vi "Modificación_Arreglos_Recetas.vi"(9 "Recetas In":T1 {"Recetas LS Electric"."Modbus LS-Electric"."Delay respuesta" min=1 max=250 format="%.0f mseg."; "Recetas LS Electric"."Modbus LS-Electric"."Formato RS485" items=["RTU 8-N-1", "RTU 8-N-2", "RTU 8-E-1", "RTU 8-O-1"]; "Recetas LS Electric"."Modbus LS-Electric"."Velocidad datos" items=["1200 bps", "2400 bps", "4800 bps", "9600 bps", "19200 bps", "38400 bps", "56 kbps", "115 kbps"]; "Recetas LS Electric"."Modbus LS-Electric"."Identificador" min=1 max=250; "Recetas LS Electric"."Motor LS-Electric 2"."Voltaje nominal" min=170 max=480 format="%.0f V"; "Recetas LS Electric"."Motor LS-Electric 2"."Potencia nominal" items=["0.2 kW", "0.4 kW", "0.75 kW", "1.1 kW", "1.5 kW", "2.2 kW", "3.0 kW", "3.7 kW", "4.0 kW", "5.5 kW", "7.5 kW", "11.kW"]; "Recetas LS Electric"."Motor LS-Electric 2"."T. Desaceleración" format="%#_g seg"; "Recetas LS Electric"."Motor LS-Electric 2"."T. Aceleración" format="%#_g seg"; "Recetas LS Electric"."Motor LS-Electric 2"."Frecuencia máxima" format="%#_g Hz"; "Recetas LS Electric"."Motor LS-Electric 2"."Frecuencia mínima" format="%#_g Hz"; "Recetas LS Electric"."Motor LS-Electric 2"."Polos" min=2 max=48; "Recetas LS Electric"."Motor LS-Electric 2"."Velocidad nominal" format="%.0f rpm"; "Recetas LS Electric"."Motor LS-Electric 2"."Corriente nominal" format="%#_g Amp"; "Recetas LS Electric"."Motor LS-Electric 2"."Corriente sin carga" format="%#_g Amp"; "Recetas LS Electric"."Motor LS-Electric 2"."Frecuencia nominal" items=["60 Hz", "50 Hz"]; "Recetas LS Electric"."Referencias LS-Electric"."Referencia velocidad 2" items=["No asignar"=0, "Analógica (AI1)"=1, "Analógica (AI2)"=2, "Analógica (AI3)"=3, "Modbus"=164, "Potenciómetro (AIU1)"=183]; "Recetas LS Electric"."Referencias LS-Electric"."Referencia arranque 2" items=["Terminales"=1, "Modbus"=10]; "Recetas LS Electric"."Referencias LS-Electric"."Referencia velocidad 1" items=["No asignar"=0, "Analógica (AI1)"=1, "Analógica (AI2)"=2, "Analógica (AI3)"=3, "Modbus"=164, "Potenciómetro (AIU1)"=183]; "Recetas LS Electric"."Referencias LS-Electric"."Referencia arranque 1" items=["Terminales"=1, "Modbus"=10]; "Recetas LS Electric"."I/O LS-Electric"."Relevador 2" items=["Modbus"=0, "FDT-1"=1, "FDT-2"=2, "FDT-3"=3, "FDT-4"=4, "Sobrecarga"=5, "Sobrevoltaje"=10, "Bajo voltaje"=11, "Sobrecalentamiento"=12, "RUN"=14, "STOP"=15, "Listo"=22]; "Recetas LS Electric"."I/O LS-Electric"."Relevador 1" items=["Modbus"=0, "FDT-1"=1, "FDT-2"=2, "FDT-3"=3, "FDT-4"=4, "Sobrecarga"=5, "Sobrevoltaje"=10, "Bajo voltaje"=11, "Sobrecalentamiento"=12, "RUN"=14, "STOP"=15, "Listo"=22]; "Recetas LS Electric"."I/O LS-Electric"."Entrada 5 (P5)" items=["No asignar"=0, "FWD"=1, "REV"=2, "Reset"=3, "Fallo auxiliar (BX)"=5, "Habilitar RUN"=13, "3 hilos"=14, "Segunda referencia"=15, "Segundo motor"=26]; "Recetas LS Electric"."I/O LS-Electric"."Entrada 4 (P4)" items=["Sin asignar"=0, "FWD"=1, "REV"=2, "Reset"=3, "Fallo auxiliar (BX)"=5, "Habilitar RUN"=13, "3 hilos"=14, "Segunda referencia"=15, "Segundo motor"=26]; "Recetas LS Electric"."I/O LS-Electric"."Entrada 3 (P3)" items=["No asignar"=0, "FWD"=1, "REV"=2, "Reset"=3, "Fallo auxiliar (BX)"=5, "Habilitar RUN"=13, "3 hilos"=14, "Segunda referencia"=15, "Segundo motor"=26]; "Recetas LS Electric"."I/O LS-Electric"."Entrada 2 (P2)" items=["No asignar"=0, "FWD"=1, "REV"=2, "Reset"=3, "Fallo auxiliar (BX)"=5, "Habilitar RUN"=13, "3 hilos"=14, "Segunda referencia"=15, "Segundo motor"=26]; "Recetas LS Electric"."I/O LS-Electric"."Entrada 1 (P1)" items=["No asignar"=0, "FWD"=1, "REV"=2, "Reset"=3, "Fallo auxiliar (BX)"=5, "Habilitar RUN"=13, "3 hilos"=14, "Segunda referencia"=15, "Segundo motor"=26]; "Recetas ABB"."Referencias ABB"."Referencia velocidad 2" items=["No asignar"=0, "Analógica (AI1)"=1, "Analógica (AI2)"=2, "Analógica (AI3)"=3, "Modbus"=164, "Potenciómetro (AIU1)"=183]; "Recetas ABB"."Referencias ABB"."Referencia arranque 2" items=["Terminales"=1, "Modbus"=10]; "Recetas ABB"."Referencias ABB"."Referencia velocidad 1" items=["No asignar"=0, "Analógica (AI1)"=1, "Analógica (AI2)"=2, "Analógica (AI3)"=3, "Modbus"=164, "Potenciómetro (AIU1)"=183]; "Recetas ABB"."Referencias ABB"."Referencia arranque 1" items=["Terminales"=1, "Modbus"=10]; "Recetas ABB"."I/O ABB"."Entrada 4 (DI4)" items=["Sin asignar"=0, "Referencia vel. 2"=1, "Referencia vel. 3"=2, "Fallo auxiliar"=12, "Reset"=13, "Entrada lógica 1"=24, "Entrada lógica 2"=25]; "Recetas ABB"."I/O ABB"."Entrada 3 (DI3)" items=["No asignar"=0, "Referencia vel. 2"=1, "Referencia vel. 3"=2, "Fallo auxiliar"=12, "Reset"=13, "Entrada lógica 1"=24, "Entrada lógica 2"=25]; "Recetas ABB"."I/O ABB"."Entrada 2 (DI2)" items=["No asignar"=0, "Referencia vel. 2"=1, "Referencia vel. 3"=2, "Fallo auxiliar"=12, "Reset"=13, "Entrada lógica 1"=24, "Entrada lógica 2"=25, "REV 2 hilos"=50, "DIR 3 hilos"=51]; "Recetas ABB"."I/O ABB"."Entrada 1 (DI1)" items=["No asignar"=0, "Referencia vel. 2"=1, "Referencia vel. 3"=2, "Fallo auxiliar"=12, "Reset"=13, "Entrada lógica 1"=24, "Entrada lógica 2"=25, "FWD 2 hilos"=48, "RUN 3 hilos"=49]; "Recetas Delta"."Referencias Delta"."Referencia velocidad 2" items=["No asignar"=0, "Analógica (AI1)"=1, "Analógica (AI2)"=2, "Analógica (AI3)"=3, "Modbus"=164, "Potenciómetro (AIU1)"=183]; "Recetas Delta"."Referencias Delta"."Referencia arranque 2" items=["Terminales"=1, "Modbus"=10]; "Recetas Delta"."Referencias Delta"."Referencia velocidad 1" items=["No asignar"=0, "Analógica (AI1)"=1, "Analógica (AI2)"=2, "Analógica (AI3)"=3, "Modbus"=164, "Potenciómetro (AIU1)"=183]; "Recetas Delta"."Referencias Delta"."Referencia arranque 1" items=["Terminales"=1, "Modbus"=10]; "Recetas Delta"."I/O Delta"."Entrada 6 (MI6)" items=["Listo/Fallo"=0, "A frecuencia"=1, "Alimentación"=2, "Sobrefrecuencia"=6, "Sobrecorriente"=7, "Sobretensión"=8, "Modbus"=13]; "Recetas Delta"."I/O Delta"."Entrada 5 (MI5)" items=["Listo/Fallo"=0, "A frecuencia"=1, "Alimentación"=2, "Sobrefrecuencia"=6, "Sobrecorriente"=7, "Sobretensión"=8, "Modbus"=13]; "Recetas Delta"."I/O Delta"."Entrada 4 (MI4)" items=["Sin asignar"=0, "Referencia vel. 2"=1, "Referencia vel. 3"=2, "Fallo auxiliar"=12, "Reset"=13, "Entrada lógica 1"=24, "Entrada lógica 2"=25]; "Recetas Delta"."I/O Delta"."Entrada 3 (MI3)" items=["No asignar"=0, "Referencia vel. 2"=1, "Referencia vel. 3"=2, "Fallo auxiliar"=12, "Reset"=13, "Entrada lógica 1"=24, "Entrada lógica 2"=25]; "Recetas Delta"."I/O Delta"."Entrada 2 (MI2)" items=["No asignar"=0, "Referencia vel. 2"=1, "Referencia vel. 3"=2, "Fallo auxiliar"=12, "Reset"=13, "Entrada lógica 1"=24, "Entrada lógica 2"=25, "REV 2 hilos"=50, "DIR 3 hilos"=51]; "Recetas Delta"."I/O Delta"."Entrada 1 (MI1)" items=["No asignar"=0, "Referencia vel. 2"=1, "Referencia vel. 3"=2, "Fallo auxiliar"=12, "Reset"=13, "Entrada lógica 1"=24, "Entrada lógica 2"=25, "FWD 2 hilos"=48, "RUN 3 hilos"=49]; "Recetas Schneider"."I/O Schneider"."Transistor" items=["Listo/Fallo"=0, "A frecuencia"=1, "Alimentación"=2, "Sobrefrecuencia"=6, "Sobrecorriente"=7, "Sobretensión"=8, "Modbus"=13]; "Recetas Schneider"."I/O Schneider"."Relevador 2 (R2)" items=["Listo/Fallo"=0, "A frecuencia"=1, "Alimentación"=2, "Sobrefrecuencia"=6, "Sobrecorriente"=7, "Sobretensión"=8, "Modbus"=13]; "Recetas Schneider"."I/O Schneider"."Relevador 1 (R1)" items=["Listo/Fallo"=0, "A frecuencia"=1, "Alimentación"=2, "Sobrefrecuencia"=6, "Sobrecorriente"=7, "Sobretensión"=8, "Modbus"=13]; "Recetas Schneider"."I/O Schneider"."Entrada 6 (DI6)" items=["Listo/Fallo"=0, "A frecuencia"=1, "Alimentación"=2, "Sobrefrecuencia"=6, "Sobrecorriente"=7, "Sobretensión"=8, "Modbus"=13]; "Recetas Schneider"."I/O Schneider"."Entrada 5 (DI5)" items=["Listo/Fallo"=0, "A frecuencia"=1, "Alimentación"=2, "Sobrefrecuencia"=6, "Sobrecorriente"=7, "Sobretensión"=8, "Modbus"=13]; "Recetas Schneider"."I/O Schneider"."Entrada 4 (DI4)" items=["Sin asignar"=0, "Referencia vel. 2"=1, "Referencia vel. 3"=2, "Fallo auxiliar"=12, "Reset"=13, "Entrada lógica 1"=24, "Entrada lógica 2"=25]; "Recetas Schneider"."I/O Schneider"."Entrada 3 (DI3)" items=["No asignar"=0, "Referencia vel. 2"=1, "Referencia vel. 3"=2, "Fallo auxiliar"=12, "Reset"=13, "Entrada lógica 1"=24, "Entrada lógica 2"=25]; "Recetas Schneider"."I/O Schneider"."Entrada 2 (DI2)" items=["No asignar"=0, "Referencia vel. 2"=1, "Referencia vel. 3"=2, "Fallo auxiliar"=12, "Reset"=13, "Entrada lógica 1"=24, "Entrada lógica 2"=25, "REV 2 hilos"=50, "DIR 3 hilos"=51]; "Recetas Schneider"."I/O Schneider"."Entrada 1 (DI1)" items=["No asignar"=0, "Referencia vel. 2"=1, "Referencia vel. 3"=2, "Fallo auxiliar"=12, "Reset"=13, "Entrada lógica 1"=24, "Entrada lógica 2"=25, "FWD 2 hilos"=48, "RUN 3 hilos"=49]; "Recetas Schneider"."Referencias Schneider"."Referencia velocidad 2" items=["No asignar"=0, "Analógica (AI1)"=1, "Analógica (AI2)"=2, "Analógica (AI3)"=3, "Modbus"=164, "Potenciómetro (AIU1)"=183]; "Recetas Schneider"."Referencias Schneider"."Referencia arranque 2" items=["Terminales"=1, "Modbus"=10]; "Recetas Schneider"."Referencias Schneider"."Referencia velocidad 1" items=["No asignar"=0, "Analógica (AI1)"=1, "Analógica (AI2)"=2, "Analógica (AI3)"=3, "Modbus"=164, "Potenciómetro (AIU1)"=183]; "Recetas Schneider"."Referencias Schneider"."Referencia arranque 1" items=["Terminales"=1, "Modbus"=10]; "Recetas Allen Bradley"."Modbus PowerFlex"."Tmp. pérdida comun." min=0.0 max=60.0 format="%#_g seg."; "Recetas Allen Bradley"."Modbus PowerFlex"."Identificador" min=1 max=247; "Recetas Allen Bradley"."Modbus PowerFlex"."Formato RS485" items=["RTU 8-N-1", "RTU 8-E-1", "RTU 8-O-1", "RTU 8-N-2", "RTU 8-E-2", "RTU 8-O-2"]; "Recetas Allen Bradley"."Modbus PowerFlex"."Acc. pérdida comun." items=["Fallo", "Paro inercia", "Paro", "Nada"]; "Recetas Allen Bradley"."Modbus PowerFlex"."Velocidad datos" items=["9600 bps", "2400 bps", "4800 bps", "9600 bps", "19200 bps", "38400 bps"]; "Recetas Allen Bradley"."Motor PowerFlex"."T. Desaleceración" format="%#_g seg"; "Recetas Allen Bradley"."Motor PowerFlex"."T. Aceleración" format="%#_g seg"; "Recetas Allen Bradley"."Motor PowerFlex"."Velocidad nominal" format="%.0f rpm"; "Recetas Allen Bradley"."Motor PowerFlex"."Voltaje nominal" format="%.0f V"; "Recetas Allen Bradley"."Motor PowerFlex"."Frecuencia nominal" format="%.0f Hz"; "Recetas Allen Bradley"."Motor PowerFlex"."Corriente sobrecarga" format="%#_g Amp"; "Recetas Allen Bradley"."Motor PowerFlex"."Corriente nominal" format="%#_g Amp"; "Recetas Allen Bradley"."Motor PowerFlex"."Polos" min=2 max=40; "Recetas Allen Bradley"."I/O PowerFlex"."Relevador" items=["Listo/Fallo"=0, "A frecuencia"=1, "Alimentación"=2, "Sobrefrecuencia"=6, "Sobrecorriente"=7, "Sobretensión"=8, "Modbus"=13]; "Recetas Allen Bradley"."I/O PowerFlex"."Entrada 6 (06)" items=["No asignar"=0, "Referencia vel. 2"=1, "Referencia vel. 3"=2, "Fallo auxiliar"=12, "Reset"=13, "Entrada lógica 1"=24, "Entrada lógica 2"=25]; "Recetas Allen Bradley"."I/O PowerFlex"."Entrada 5 (05)" items=["No asignar"=0, "Referencia vel. 2"=1, "Referencia vel. 3"=2, "Fallo auxiliar"=12, "Reset"=13, "Entrada lógica 1"=24, "Entrada lógica 2"=25]; "Recetas Allen Bradley"."I/O PowerFlex"."Entrada 3 (03)" items=["No asignar"=0, "Referencia vel. 2"=1, "Referencia vel. 3"=2, "Fallo auxiliar"=12, "Reset"=13, "Entrada lógica 1"=24, "Entrada lógica 2"=25, "REV 2 hilos"=50, "DIR 3 hilos"=51]; "Recetas Allen Bradley"."I/O PowerFlex"."Entrada 2 (02)" items=["No asignar"=0, "Referencia vel. 2"=1, "Referencia vel. 3"=2, "Fallo auxiliar"=12, "Reset"=13, "Entrada lógica 1"=24, "Entrada lógica 2"=25, "FWD 2 hilos"=48, "RUN 3 hilos"=49]; "Recetas Allen Bradley"."Referencias PowerFlex"."Referencia velocidad 2" items=["Potenciómetro"=1, "Teclado"=2, "Modbus"=3, "Analógica (0-10V)"=5, "Analógica (4-20mA)"=6]; "Recetas Allen Bradley"."Referencias PowerFlex"."Referencia arranque 2" items=["Teclado"=1, "Terminales"=2, "Modbus"=3]; "Recetas Allen Bradley"."Referencias PowerFlex"."Referencia velocidad 1" items=["Potenciómetro"=1, "Teclado"=2, "Modbus"=3, "Analógica (0-10V)"=5, "Analógica (4-20mA)"=6]; "Recetas Allen Bradley"."Referencias PowerFlex"."Referencia arranque 1" items=["Teclado"=1, "Terminales"=2, "Modbus"=3]}, 10 "Fabricante":u32, 11 "Índice":u32) -> (3 "Recetas Out":T1 {"Recetas LS Electric"."Modbus LS-Electric"."Delay respuesta" min=1 max=250 format="%.0f mseg."; "Recetas LS Electric"."Modbus LS-Electric"."Formato RS485" items=["RTU 8-N-1", "RTU 8-N-2", "RTU 8-E-1", "RTU 8-O-1"]; "Recetas LS Electric"."Modbus LS-Electric"."Velocidad datos" items=["1200 bps", "2400 bps", "4800 bps", "9600 bps", "19200 bps", "38400 bps", "56 kbps", "115 kbps"]; "Recetas LS Electric"."Modbus LS-Electric"."Identificador" min=1 max=250; "Recetas LS Electric"."Motor LS-Electric 2"."Voltaje nominal" min=170 max=480 format="%.0f V"; "Recetas LS Electric"."Motor LS-Electric 2"."Potencia nominal" items=["0.2 kW", "0.4 kW", "0.75 kW", "1.1 kW", "1.5 kW", "2.2 kW", "3.0 kW", "3.7 kW", "4.0 kW", "5.5 kW", "7.5 kW", "11.kW"]; "Recetas LS Electric"."Motor LS-Electric 2"."T. Desaceleración" format="%#_g seg"; "Recetas LS Electric"."Motor LS-Electric 2"."T. Aceleración" format="%#_g seg"; "Recetas LS Electric"."Motor LS-Electric 2"."Frecuencia máxima" format="%#_g Hz"; "Recetas LS Electric"."Motor LS-Electric 2"."Frecuencia mínima" format="%#_g Hz"; "Recetas LS Electric"."Motor LS-Electric 2"."Polos" min=2 max=48; "Recetas LS Electric"."Motor LS-Electric 2"."Velocidad nominal" format="%.0f rpm"; "Recetas LS Electric"."Motor LS-Electric 2"."Corriente nominal" format="%#_g Amp"; "Recetas LS Electric"."Motor LS-Electric 2"."Corriente sin carga" format="%#_g Amp"; "Recetas LS Electric"."Motor LS-Electric 2"."Frecuencia nominal" items=["60 Hz", "50 Hz"]; "Recetas LS Electric"."Referencias LS-Electric"."Referencia velocidad 2" items=["No asignar"=0, "Analógica (AI1)"=1, "Analógica (AI2)"=2, "Analógica (AI3)"=3, "Modbus"=164, "Potenciómetro (AIU1)"=183]; "Recetas LS Electric"."Referencias LS-Electric"."Referencia arranque 2" items=["Terminales"=1, "Modbus"=10]; "Recetas LS Electric"."Referencias LS-Electric"."Referencia velocidad 1" items=["No asignar"=0, "Analógica (AI1)"=1, "Analógica (AI2)"=2, "Analógica (AI3)"=3, "Modbus"=164, "Potenciómetro (AIU1)"=183]; "Recetas LS Electric"."Referencias LS-Electric"."Referencia arranque 1" items=["Terminales"=1, "Modbus"=10]; "Recetas LS Electric"."I/O LS-Electric"."Relevador 2" items=["Modbus"=0, "FDT-1"=1, "FDT-2"=2, "FDT-3"=3, "FDT-4"=4, "Sobrecarga"=5, "Sobrevoltaje"=10, "Bajo voltaje"=11, "Sobrecalentamiento"=12, "RUN"=14, "STOP"=15, "Listo"=22]; "Recetas LS Electric"."I/O LS-Electric"."Relevador 1" items=["Modbus"=0, "FDT-1"=1, "FDT-2"=2, "FDT-3"=3, "FDT-4"=4, "Sobrecarga"=5, "Sobrevoltaje"=10, "Bajo voltaje"=11, "Sobrecalentamiento"=12, "RUN"=14, "STOP"=15, "Listo"=22]; "Recetas LS Electric"."I/O LS-Electric"."Entrada 5 (P5)" items=["No asignar"=0, "FWD"=1, "REV"=2, "Reset"=3, "Fallo auxiliar (BX)"=5, "Habilitar RUN"=13, "3 hilos"=14, "Segunda referencia"=15, "Segundo motor"=26]; "Recetas LS Electric"."I/O LS-Electric"."Entrada 4 (P4)" items=["Sin asignar"=0, "FWD"=1, "REV"=2, "Reset"=3, "Fallo auxiliar (BX)"=5, "Habilitar RUN"=13, "3 hilos"=14, "Segunda referencia"=15, "Segundo motor"=26]; "Recetas LS Electric"."I/O LS-Electric"."Entrada 3 (P3)" items=["No asignar"=0, "FWD"=1, "REV"=2, "Reset"=3, "Fallo auxiliar (BX)"=5, "Habilitar RUN"=13, "3 hilos"=14, "Segunda referencia"=15, "Segundo motor"=26]; "Recetas LS Electric"."I/O LS-Electric"."Entrada 2 (P2)" items=["No asignar"=0, "FWD"=1, "REV"=2, "Reset"=3, "Fallo auxiliar (BX)"=5, "Habilitar RUN"=13, "3 hilos"=14, "Segunda referencia"=15, "Segundo motor"=26]; "Recetas LS Electric"."I/O LS-Electric"."Entrada 1 (P1)" items=["No asignar"=0, "FWD"=1, "REV"=2, "Reset"=3, "Fallo auxiliar (BX)"=5, "Habilitar RUN"=13, "3 hilos"=14, "Segunda referencia"=15, "Segundo motor"=26]; "Recetas ABB"."Referencias ABB"."Referencia velocidad 2" items=["No asignar"=0, "Analógica (AI1)"=1, "Analógica (AI2)"=2, "Analógica (AI3)"=3, "Modbus"=164, "Potenciómetro (AIU1)"=183]; "Recetas ABB"."Referencias ABB"."Referencia arranque 2" items=["Terminales"=1, "Modbus"=10]; "Recetas ABB"."Referencias ABB"."Referencia velocidad 1" items=["No asignar"=0, "Analógica (AI1)"=1, "Analógica (AI2)"=2, "Analógica (AI3)"=3, "Modbus"=164, "Potenciómetro (AIU1)"=183]; "Recetas ABB"."Referencias ABB"."Referencia arranque 1" items=["Terminales"=1, "Modbus"=10]; "Recetas ABB"."I/O ABB"."Entrada 4 (DI4)" items=["Sin asignar"=0, "Referencia vel. 2"=1, "Referencia vel. 3"=2, "Fallo auxiliar"=12, "Reset"=13, "Entrada lógica 1"=24, "Entrada lógica 2"=25]; "Recetas ABB"."I/O ABB"."Entrada 3 (DI3)" items=["No asignar"=0, "Referencia vel. 2"=1, "Referencia vel. 3"=2, "Fallo auxiliar"=12, "Reset"=13, "Entrada lógica 1"=24, "Entrada lógica 2"=25]; "Recetas ABB"."I/O ABB"."Entrada 2 (DI2)" items=["No asignar"=0, "Referencia vel. 2"=1, "Referencia vel. 3"=2, "Fallo auxiliar"=12, "Reset"=13, "Entrada lógica 1"=24, "Entrada lógica 2"=25, "REV 2 hilos"=50, "DIR 3 hilos"=51]; "Recetas ABB"."I/O ABB"."Entrada 1 (DI1)" items=["No asignar"=0, "Referencia vel. 2"=1, "Referencia vel. 3"=2, "Fallo auxiliar"=12, "Reset"=13, "Entrada lógica 1"=24, "Entrada lógica 2"=25, "FWD 2 hilos"=48, "RUN 3 hilos"=49]; "Recetas Delta"."Referencias Delta"."Referencia velocidad 2" items=["No asignar"=0, "Analógica (AI1)"=1, "Analógica (AI2)"=2, "Analógica (AI3)"=3, "Modbus"=164, "Potenciómetro (AIU1)"=183]; "Recetas Delta"."Referencias Delta"."Referencia arranque 2" items=["Terminales"=1, "Modbus"=10]; "Recetas Delta"."Referencias Delta"."Referencia velocidad 1" items=["No asignar"=0, "Analógica (AI1)"=1, "Analógica (AI2)"=2, "Analógica (AI3)"=3, "Modbus"=164, "Potenciómetro (AIU1)"=183]; "Recetas Delta"."Referencias Delta"."Referencia arranque 1" items=["Terminales"=1, "Modbus"=10]; "Recetas Delta"."I/O Delta"."Entrada 6 (MI6)" items=["Listo/Fallo"=0, "A frecuencia"=1, "Alimentación"=2, "Sobrefrecuencia"=6, "Sobrecorriente"=7, "Sobretensión"=8, "Modbus"=13]; "Recetas Delta"."I/O Delta"."Entrada 5 (MI5)" items=["Listo/Fallo"=0, "A frecuencia"=1, "Alimentación"=2, "Sobrefrecuencia"=6, "Sobrecorriente"=7, "Sobretensión"=8, "Modbus"=13]; "Recetas Delta"."I/O Delta"."Entrada 4 (MI4)" items=["Sin asignar"=0, "Referencia vel. 2"=1, "Referencia vel. 3"=2, "Fallo auxiliar"=12, "Reset"=13, "Entrada lógica 1"=24, "Entrada lógica 2"=25]; "Recetas Delta"."I/O Delta"."Entrada 3 (MI3)" items=["No asignar"=0, "Referencia vel. 2"=1, "Referencia vel. 3"=2, "Fallo auxiliar"=12, "Reset"=13, "Entrada lógica 1"=24, "Entrada lógica 2"=25]; "Recetas Delta"."I/O Delta"."Entrada 2 (MI2)" items=["No asignar"=0, "Referencia vel. 2"=1, "Referencia vel. 3"=2, "Fallo auxiliar"=12, "Reset"=13, "Entrada lógica 1"=24, "Entrada lógica 2"=25, "REV 2 hilos"=50, "DIR 3 hilos"=51]; "Recetas Delta"."I/O Delta"."Entrada 1 (MI1)" items=["No asignar"=0, "Referencia vel. 2"=1, "Referencia vel. 3"=2, "Fallo auxiliar"=12, "Reset"=13, "Entrada lógica 1"=24, "Entrada lógica 2"=25, "FWD 2 hilos"=48, "RUN 3 hilos"=49]; "Recetas Schneider"."I/O Schneider"."Transistor" items=["Listo/Fallo"=0, "A frecuencia"=1, "Alimentación"=2, "Sobrefrecuencia"=6, "Sobrecorriente"=7, "Sobretensión"=8, "Modbus"=13]; "Recetas Schneider"."I/O Schneider"."Relevador 2 (R2)" items=["Listo/Fallo"=0, "A frecuencia"=1, "Alimentación"=2, "Sobrefrecuencia"=6, "Sobrecorriente"=7, "Sobretensión"=8, "Modbus"=13]; "Recetas Schneider"."I/O Schneider"."Relevador 1 (R1)" items=["Listo/Fallo"=0, "A frecuencia"=1, "Alimentación"=2, "Sobrefrecuencia"=6, "Sobrecorriente"=7, "Sobretensión"=8, "Modbus"=13]; "Recetas Schneider"."I/O Schneider"."Entrada 6 (DI6)" items=["Listo/Fallo"=0, "A frecuencia"=1, "Alimentación"=2, "Sobrefrecuencia"=6, "Sobrecorriente"=7, "Sobretensión"=8, "Modbus"=13]; "Recetas Schneider"."I/O Schneider"."Entrada 5 (DI5)" items=["Listo/Fallo"=0, "A frecuencia"=1, "Alimentación"=2, "Sobrefrecuencia"=6, "Sobrecorriente"=7, "Sobretensión"=8, "Modbus"=13]; "Recetas Schneider"."I/O Schneider"."Entrada 4 (DI4)" items=["Sin asignar"=0, "Referencia vel. 2"=1, "Referencia vel. 3"=2, "Fallo auxiliar"=12, "Reset"=13, "Entrada lógica 1"=24, "Entrada lógica 2"=25]; "Recetas Schneider"."I/O Schneider"."Entrada 3 (DI3)" items=["No asignar"=0, "Referencia vel. 2"=1, "Referencia vel. 3"=2, "Fallo auxiliar"=12, "Reset"=13, "Entrada lógica 1"=24, "Entrada lógica 2"=25]; "Recetas Schneider"."I/O Schneider"."Entrada 2 (DI2)" items=["No asignar"=0, "Referencia vel. 2"=1, "Referencia vel. 3"=2, "Fallo auxiliar"=12, "Reset"=13, "Entrada lógica 1"=24, "Entrada lógica 2"=25, "REV 2 hilos"=50, "DIR 3 hilos"=51]; "Recetas Schneider"."I/O Schneider"."Entrada 1 (DI1)" items=["No asignar"=0, "Referencia vel. 2"=1, "Referencia vel. 3"=2, "Fallo auxiliar"=12, "Reset"=13, "Entrada lógica 1"=24, "Entrada lógica 2"=25, "FWD 2 hilos"=48, "RUN 3 hilos"=49]; "Recetas Schneider"."Referencias Schneider"."Referencia velocidad 2" items=["No asignar"=0, "Analógica (AI1)"=1, "Analógica (AI2)"=2, "Analógica (AI3)"=3, "Modbus"=164, "Potenciómetro (AIU1)"=183]; "Recetas Schneider"."Referencias Schneider"."Referencia arranque 2" items=["Terminales"=1, "Modbus"=10]; "Recetas Schneider"."Referencias Schneider"."Referencia velocidad 1" items=["No asignar"=0, "Analógica (AI1)"=1, "Analógica (AI2)"=2, "Analógica (AI3)"=3, "Modbus"=164, "Potenciómetro (AIU1)"=183]; "Recetas Schneider"."Referencias Schneider"."Referencia arranque 1" items=["Terminales"=1, "Modbus"=10]; "Recetas Allen Bradley"."Modbus PowerFlex"."Tmp. pérdida comun." min=0.0 max=60.0 format="%#_g seg."; "Recetas Allen Bradley"."Modbus PowerFlex"."Identificador" min=1 max=247; "Recetas Allen Bradley"."Modbus PowerFlex"."Formato RS485" items=["RTU 8-N-1", "RTU 8-E-1", "RTU 8-O-1", "RTU 8-N-2", "RTU 8-E-2", "RTU 8-O-2"]; "Recetas Allen Bradley"."Modbus PowerFlex"."Acc. pérdida comun." items=["Fallo", "Paro inercia", "Paro", "Nada"]; "Recetas Allen Bradley"."Modbus PowerFlex"."Velocidad datos" items=["9600 bps", "2400 bps", "4800 bps", "9600 bps", "19200 bps", "38400 bps"]; "Recetas Allen Bradley"."Motor PowerFlex"."T. Desaleceración" format="%#_g seg"; "Recetas Allen Bradley"."Motor PowerFlex"."T. Aceleración" format="%#_g seg"; "Recetas Allen Bradley"."Motor PowerFlex"."Velocidad nominal" format="%.0f rpm"; "Recetas Allen Bradley"."Motor PowerFlex"."Voltaje nominal" format="%.0f V"; "Recetas Allen Bradley"."Motor PowerFlex"."Frecuencia nominal" format="%.0f Hz"; "Recetas Allen Bradley"."Motor PowerFlex"."Corriente sobrecarga" format="%#_g Amp"; "Recetas Allen Bradley"."Motor PowerFlex"."Corriente nominal" format="%#_g Amp"; "Recetas Allen Bradley"."Motor PowerFlex"."Polos" min=2 max=40; "Recetas Allen Bradley"."I/O PowerFlex"."Relevador" items=["Listo/Fallo"=0, "A frecuencia"=1, "Alimentación"=2, "Sobrefrecuencia"=6, "Sobrecorriente"=7, "Sobretensión"=8, "Modbus"=13]; "Recetas Allen Bradley"."I/O PowerFlex"."Entrada 6 (06)" items=["No asignar"=0, "Referencia vel. 2"=1, "Referencia vel. 3"=2, "Fallo auxiliar"=12, "Reset"=13, "Entrada lógica 1"=24, "Entrada lógica 2"=25]; "Recetas Allen Bradley"."I/O PowerFlex"."Entrada 5 (05)" items=["No asignar"=0, "Referencia vel. 2"=1, "Referencia vel. 3"=2, "Fallo auxiliar"=12, "Reset"=13, "Entrada lógica 1"=24, "Entrada lógica 2"=25]; "Recetas Allen Bradley"."I/O PowerFlex"."Entrada 3 (03)" items=["No asignar"=0, "Referencia vel. 2"=1, "Referencia vel. 3"=2, "Fallo auxiliar"=12, "Reset"=13, "Entrada lógica 1"=24, "Entrada lógica 2"=25, "REV 2 hilos"=50, "DIR 3 hilos"=51]; "Recetas Allen Bradley"."I/O PowerFlex"."Entrada 2 (02)" items=["No asignar"=0, "Referencia vel. 2"=1, "Referencia vel. 3"=2, "Fallo auxiliar"=12, "Reset"=13, "Entrada lógica 1"=24, "Entrada lógica 2"=25, "FWD 2 hilos"=48, "RUN 3 hilos"=49]; "Recetas Allen Bradley"."Referencias PowerFlex"."Referencia velocidad 2" items=["Potenciómetro"=1, "Teclado"=2, "Modbus"=3, "Analógica (0-10V)"=5, "Analógica (4-20mA)"=6]; "Recetas Allen Bradley"."Referencias PowerFlex"."Referencia arranque 2" items=["Teclado"=1, "Terminales"=2, "Modbus"=3]; "Recetas Allen Bradley"."Referencias PowerFlex"."Referencia velocidad 1" items=["Potenciómetro"=1, "Teclado"=2, "Modbus"=3, "Analógica (0-10V)"=5, "Analógica (4-20mA)"=6]; "Recetas Allen Bradley"."Referencias PowerFlex"."Referencia arranque 1" items=["Teclado"=1, "Terminales"=2, "Modbus"=3]})   [LabVIEW 2013]
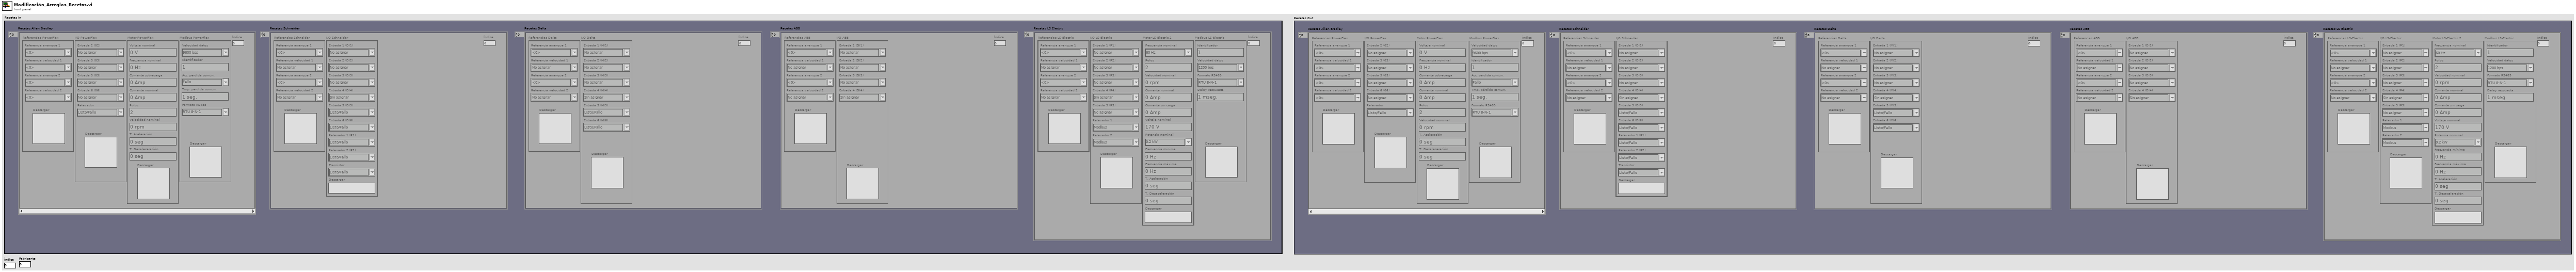
[diagram p1: front panel]
types:
  T1 = cluster{"Recetas Allen Bradley":cluster{"Referencias PowerFlex":cluster{"Referencia arranque 1":u16, "Referencia velocidad 1":u16, "Referencia arranque 2":u16, "Referencia velocidad 2":u16, "Descargar":bool}, "I/O PowerFlex":cluster{"Entrada 2 (02)":u16, "Entrada 3 (03)":u16, "Entrada 5 (05)":u16, "Entrada 6 (06)":u16, "Relevador":u16, "Descargar":bool}, "Motor PowerFlex":cluster{"Voltaje nominal":u16, "Frecuencia nominal":u16, "Corriente sobrecarga":dbl, "Corriente nominal":dbl, "Polos":u16, "Velocidad nominal":u16, "T. Aceleración":dbl, "T. Desaleceración":dbl, "Descargar":bool}, "Modbus PowerFlex":cluster{"Velocidad datos":u16, "Identificador":u16, "Acc. pérdida comun.":u16, "Tmp. pérdida comun.":dbl, "Formato RS485":u16, "Descargar":bool}, "Índice":u32}[], "Recetas Schneider":cluster{"Referencias Schneider":cluster{"Referencia arranque 1":u16, "Referencia velocidad 1":u16, "Referencia arranque 2":u16, "Referencia velocidad 2":u16, "Descargar":bool}, "I/O Schneider":cluster{"Entrada 1 (DI1)":u16, "Entrada 2 (DI2)":u16, "Entrada 3 (DI3)":u16, "Entrada 4 (DI4)":u16, "Entrada 5 (DI5)":u16, "Entrada 6 (DI6)":u16, "Relevador 1 (R1)":u16, "Relevador 2 (R2)":u16, "Transistor":u16, "Descargar":bool}, "Índice":u32}[], "Recetas Delta":cluster{"Referencias Delta":cluster{"Referencia arranque 1":u16, "Referencia velocidad 1":u16, "Referencia arranque 2":u16, "Referencia velocidad 2":u16, "Descargar":bool}, "I/O Delta":cluster{"Entrada 1 (MI1)":u16, "Entrada 2 (MI2)":u16, "Entrada 3 (MI3)":u16, "Entrada 4 (MI4)":u16, "Entrada 5 (MI5)":u16, "Entrada 6 (MI6)":u16, "Descargar":bool}, "Índice":u32}[], "Recetas ABB":cluster{"Referencias ABB":cluster{"Referencia arranque 1":u16, "Referencia velocidad 1":u16, "Referencia arranque 2":u16, "Referencia velocidad 2":u16, "Descargar":bool}, "I/O ABB":cluster{"Entrada 1 (DI1)":u16, "Entrada 2 (DI2)":u16, "Entrada 3 (DI3)":u16, "Entrada 4 (DI4)":u16, "Descargar":bool}, "Índice":u32}[], "Recetas LS Electric":cluster{"Referencias LS-Electric":cluster{"Referencia arranque 1":u16, "Referencia velocidad 1":u16, "Referencia arranque 2":u16, "Referencia velocidad 2":u16, "Descargar":bool}, "I/O LS-Electric":cluster{"Entrada 1 (P1)":u16, "Entrada 2 (P2)":u16, "Entrada 3 (P3)":u16, "Entrada 4 (P4)":u16, "Entrada 5 (P5)":u16, "Relevador 1":u16, "Relevador 2":u16, "Descargar":bool}, "Motor LS-Electric 2":cluster{"Frecuencia nominal":u16, "Polos":u16, "Velocidad nominal":u16, "Corriente nominal":dbl, "Corriente sin carga":dbl, "Voltaje nominal":u16, "Potencia nominal":u16, "Frecuencia mínima":dbl, "Frecuencia máxima":dbl, "T. Aceleración":dbl, "T. Desaceleración":dbl, "Descargar":bool}, "Modbus LS-Electric":cluster{"Identificador":u16, "Velocidad datos":u16, "Formato RS485":u16, "Delay respuesta":u16, "Descargar":bool}, "Índice":u32}[]}
  T2 = cluster{"Referencias PowerFlex":cluster{"Referencia arranque 1":u16, "Referencia velocidad 1":u16, "Referencia arranque 2":u16, "Referencia velocidad 2":u16, "Descargar":bool}, "I/O PowerFlex":cluster{"Entrada 2 (02)":u16, "Entrada 3 (03)":u16, "Entrada 5 (05)":u16, "Entrada 6 (06)":u16, "Relevador":u16, "Descargar":bool}, "Motor PowerFlex":cluster{"Voltaje nominal":u16, "Frecuencia nominal":u16, "Corriente sobrecarga":dbl, "Corriente nominal":dbl, "Polos":u16, "Velocidad nominal":u16, "T. Aceleración":dbl, "T. Desaleceración":dbl, "Descargar":bool}, "Modbus PowerFlex":cluster{"Velocidad datos":u16, "Identificador":u16, "Acc. pérdida comun.":u16, "Tmp. pérdida comun.":dbl, "Formato RS485":u16, "Descargar":bool}, "Índice":u32}[]
  T3 = cluster{"Referencias Schneider":cluster{"Referencia arranque 1":u16, "Referencia velocidad 1":u16, "Referencia arranque 2":u16, "Referencia velocidad 2":u16, "Descargar":bool}, "I/O Schneider":cluster{"Entrada 1 (DI1)":u16, "Entrada 2 (DI2)":u16, "Entrada 3 (DI3)":u16, "Entrada 4 (DI4)":u16, "Entrada 5 (DI5)":u16, "Entrada 6 (DI6)":u16, "Relevador 1 (R1)":u16, "Relevador 2 (R2)":u16, "Transistor":u16, "Descargar":bool}, "Índice":u32}[]
  T4 = cluster{"Referencias Delta":cluster{"Referencia arranque 1":u16, "Referencia velocidad 1":u16, "Referencia arranque 2":u16, "Referencia velocidad 2":u16, "Descargar":bool}, "I/O Delta":cluster{"Entrada 1 (MI1)":u16, "Entrada 2 (MI2)":u16, "Entrada 3 (MI3)":u16, "Entrada 4 (MI4)":u16, "Entrada 5 (MI5)":u16, "Entrada 6 (MI6)":u16, "Descargar":bool}, "Índice":u32}[]
  T5 = cluster{"Referencias ABB":cluster{"Referencia arranque 1":u16, "Referencia velocidad 1":u16, "Referencia arranque 2":u16, "Referencia velocidad 2":u16, "Descargar":bool}, "I/O ABB":cluster{"Entrada 1 (DI1)":u16, "Entrada 2 (DI2)":u16, "Entrada 3 (DI3)":u16, "Entrada 4 (DI4)":u16, "Descargar":bool}, "Índice":u32}[]
  T6 = cluster{"Referencias LS-Electric":cluster{"Referencia arranque 1":u16, "Referencia velocidad 1":u16, "Referencia arranque 2":u16, "Referencia velocidad 2":u16, "Descargar":bool}, "I/O LS-Electric":cluster{"Entrada 1 (P1)":u16, "Entrada 2 (P2)":u16, "Entrada 3 (P3)":u16, "Entrada 4 (P4)":u16, "Entrada 5 (P5)":u16, "Relevador 1":u16, "Relevador 2":u16, "Descargar":bool}, "Motor LS-Electric 2":cluster{"Frecuencia nominal":u16, "Polos":u16, "Velocidad nominal":u16, "Corriente nominal":dbl, "Corriente sin carga":dbl, "Voltaje nominal":u16, "Potencia nominal":u16, "Frecuencia mínima":dbl, "Frecuencia máxima":dbl, "T. Aceleración":dbl, "T. Desaceleración":dbl, "Descargar":bool}, "Modbus LS-Electric":cluster{"Identificador":u16, "Velocidad datos":u16, "Formato RS485":u16, "Delay respuesta":u16, "Descargar":bool}, "Índice":u32}[]
  T7 = cluster{"Referencias PowerFlex":cluster{"Referencia arranque 1":u16, "Referencia velocidad 1":u16, "Referencia arranque 2":u16, "Referencia velocidad 2":u16, "Descargar":bool}, "I/O PowerFlex":cluster{"Entrada 2 (02)":u16, "Entrada 3 (03)":u16, "Entrada 5 (05)":u16, "Entrada 6 (06)":u16, "Relevador":u16, "Descargar":bool}, "Motor PowerFlex":cluster{"Voltaje nominal":u16, "Frecuencia nominal":u16, "Corriente sobrecarga":dbl, "Corriente nominal":dbl, "Polos":u16, "Velocidad nominal":u16, "T. Aceleración":dbl, "T. Desaleceración":dbl, "Descargar":bool}, "Modbus PowerFlex":cluster{"Velocidad datos":u16, "Identificador":u16, "Acc. pérdida comun.":u16, "Tmp. pérdida comun.":dbl, "Formato RS485":u16, "Descargar":bool}, "Índice":u32}
  T8 = cluster{"Referencias Schneider":cluster{"Referencia arranque 1":u16, "Referencia velocidad 1":u16, "Referencia arranque 2":u16, "Referencia velocidad 2":u16, "Descargar":bool}, "I/O Schneider":cluster{"Entrada 1 (DI1)":u16, "Entrada 2 (DI2)":u16, "Entrada 3 (DI3)":u16, "Entrada 4 (DI4)":u16, "Entrada 5 (DI5)":u16, "Entrada 6 (DI6)":u16, "Relevador 1 (R1)":u16, "Relevador 2 (R2)":u16, "Transistor":u16, "Descargar":bool}, "Índice":u32}
  T9 = cluster{"Referencias Delta":cluster{"Referencia arranque 1":u16, "Referencia velocidad 1":u16, "Referencia arranque 2":u16, "Referencia velocidad 2":u16, "Descargar":bool}, "I/O Delta":cluster{"Entrada 1 (MI1)":u16, "Entrada 2 (MI2)":u16, "Entrada 3 (MI3)":u16, "Entrada 4 (MI4)":u16, "Entrada 5 (MI5)":u16, "Entrada 6 (MI6)":u16, "Descargar":bool}, "Índice":u32}
  T10 = cluster{"Referencias ABB":cluster{"Referencia arranque 1":u16, "Referencia velocidad 1":u16, "Referencia arranque 2":u16, "Referencia velocidad 2":u16, "Descargar":bool}, "I/O ABB":cluster{"Entrada 1 (DI1)":u16, "Entrada 2 (DI2)":u16, "Entrada 3 (DI3)":u16, "Entrada 4 (DI4)":u16, "Descargar":bool}, "Índice":u32}
  T11 = cluster{"Referencias LS-Electric":cluster{"Referencia arranque 1":u16, "Referencia velocidad 1":u16, "Referencia arranque 2":u16, "Referencia velocidad 2":u16, "Descargar":bool}, "I/O LS-Electric":cluster{"Entrada 1 (P1)":u16, "Entrada 2 (P2)":u16, "Entrada 3 (P3)":u16, "Entrada 4 (P4)":u16, "Entrada 5 (P5)":u16, "Relevador 1":u16, "Relevador 2":u16, "Descargar":bool}, "Motor LS-Electric 2":cluster{"Frecuencia nominal":u16, "Polos":u16, "Velocidad nominal":u16, "Corriente nominal":dbl, "Corriente sin carga":dbl, "Voltaje nominal":u16, "Potencia nominal":u16, "Frecuencia mínima":dbl, "Frecuencia máxima":dbl, "T. Aceleración":dbl, "T. Desaceleración":dbl, "Descargar":bool}, "Modbus LS-Electric":cluster{"Identificador":u16, "Velocidad datos":u16, "Formato RS485":u16, "Delay respuesta":u16, "Descargar":bool}, "Índice":u32}
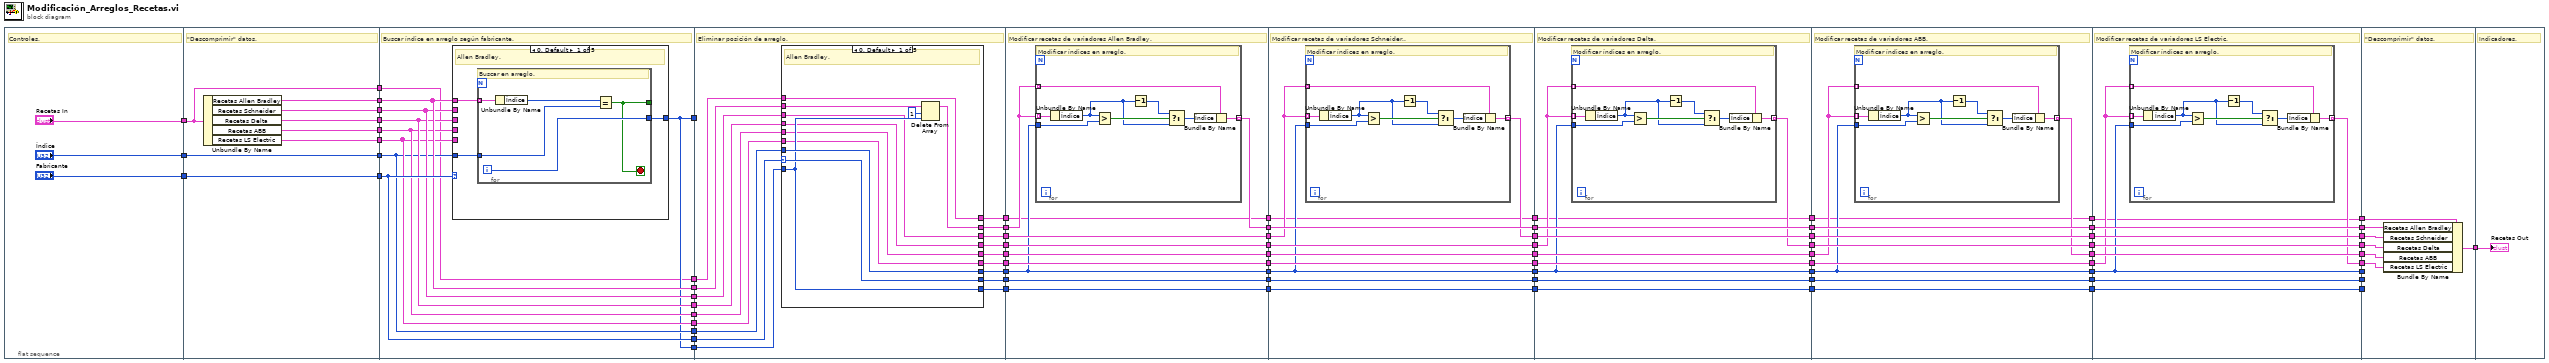
[diagram p0: block diagram]
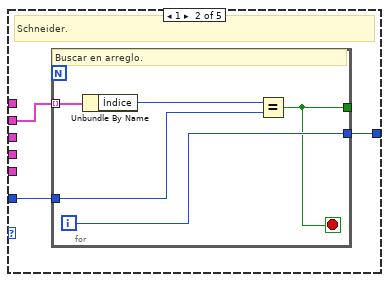
[diagram p2: hidden frame]
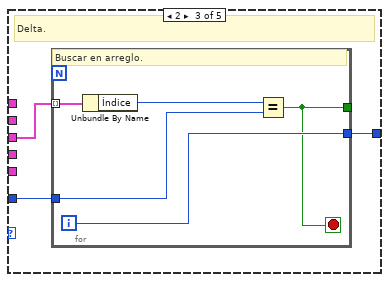
[diagram p3: hidden frame]
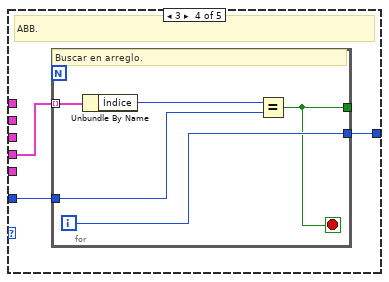
[diagram p4: hidden frame]
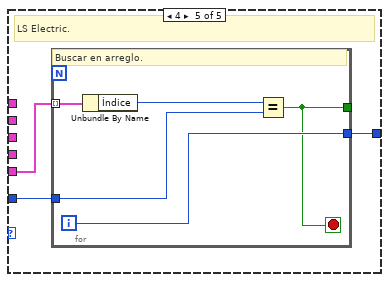
[diagram p5: hidden frame]
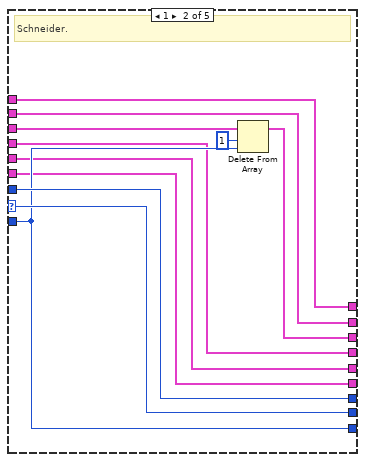
[diagram p6: hidden frame]
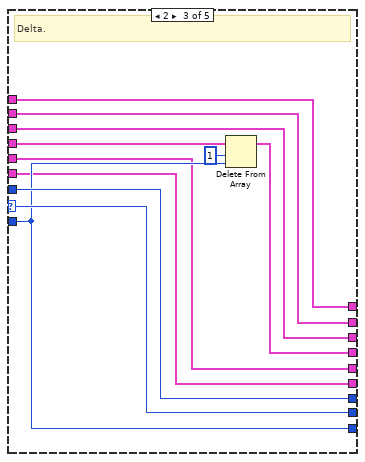
[diagram p7: hidden frame]
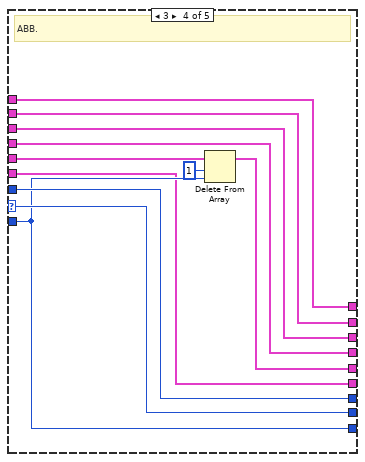
[diagram p8: hidden frame]
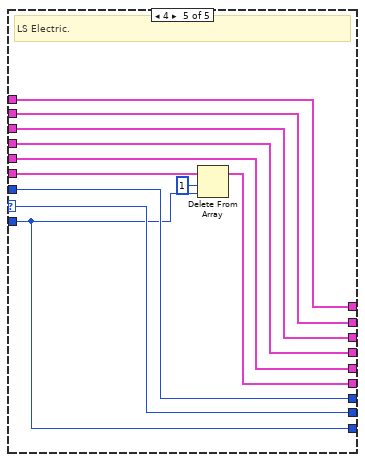
[diagram p9: hidden frame]
diagram:
  n1 = flat-sequence {
    tunnel: ["Recetas In"] -> w76
    tunnel: ["Fabricante"] -> w75
    tunnel: ["Índice"] -> w73
    tunnel: w76 -> [w80]
    tunnel: w75 -> [w81]
    tunnel: [w82] -> w74
    tunnel: w73 -> [w82]
    tunnel: [w87] -> w72
    tunnel: [w86] -> w71
    tunnel: [w85] -> w70
    tunnel: [w84] -> w69
    tunnel: [w83] -> w68
    tunnel: [w81] -> w67
    tunnel: [w80] -> w9
    tunnel: w74 -> [w90]
    tunnel: w72 -> [w95]
    tunnel: w71 -> [w94]
    tunnel: w70 -> [w93]
    tunnel: w69 -> [w92]
    tunnel: w68 -> [w91]
    tunnel: w67 -> [w96]
    tunnel: [w89] -> w66
    tunnel: [w96] -> w65
    tunnel: [w95] -> w64
    tunnel: [w94] -> w63
    tunnel: [w93] -> w62
    tunnel: [w92] -> w61
    tunnel: [w91] -> w60
    tunnel: [w90] -> w59
    tunnel: [w89] -> w58
    tunnel: w9 -> [w88]
    tunnel: [w88] -> w8
    tunnel: w66 -> [_]
    tunnel: w65 -> [w154]
    tunnel: w64 -> [w153]
    tunnel: w63 -> [w151]
    tunnel: w62 -> [w149]
    tunnel: w61 -> [w147]
    tunnel: w60 -> [w145]
    tunnel: w59 -> [w141]
    tunnel: w58 -> [w139]
    tunnel: [w152] -> w57
    tunnel: [w150] -> w56
    tunnel: [w148] -> w55
    tunnel: [w146] -> w54
    tunnel: [w144] -> w53
    tunnel: [w143] -> w52
    tunnel: [w142] -> w51
    tunnel: [w140] -> w50
    tunnel: w8 -> [w138]
    tunnel: [w137] -> w7
    tunnel: w57 -> [w212]
    tunnel: w56 -> [w214]
    tunnel: w55 -> [w215]
    tunnel: w54 -> [w216]
    tunnel: w53 -> [w217]
    tunnel: w52 -> [w213]
    tunnel: w51 -> [w218]
    tunnel: w50 -> [w219]
    tunnel: [w219] -> w49
    tunnel: [w218] -> w48
    tunnel: [w213] -> w47
    tunnel: [w217] -> w46
    tunnel: [w216] -> w45
    tunnel: [w215] -> w44
    tunnel: [w214] -> w43
    tunnel: [w211] -> w42
    tunnel: w7 -> [w210]
    tunnel: [w210] -> w6
    tunnel: w49 -> [w237]
    tunnel: w48 -> [w236]
    tunnel: w47 -> [w231]
    tunnel: w46 -> [w235]
    tunnel: w45 -> [w234]
    tunnel: w44 -> [w233]
    tunnel: w43 -> [w230]
    tunnel: w42 -> [w232]
    tunnel: [w237] -> w41
    tunnel: [w236] -> w40
    tunnel: [w231] -> w39
    tunnel: [w235] -> w38
    tunnel: [w234] -> w37
    tunnel: [w233] -> w36
    tunnel: [w229] -> w35
    tunnel: [w232] -> w34
    tunnel: w6 -> [w228]
    tunnel: [w228] -> w5
    tunnel: w41 -> [w255]
    tunnel: w40 -> [w254]
    tunnel: w39 -> [w249]
    tunnel: w38 -> [w253]
    tunnel: w37 -> [w252]
    tunnel: w36 -> [w248]
    tunnel: w35 -> [w251]
    tunnel: w34 -> [w250]
    tunnel: [w255] -> w33
    tunnel: [w254] -> w32
    tunnel: [w249] -> w31
    tunnel: [w253] -> w30
    tunnel: [w252] -> w29
    tunnel: [w247] -> w28
    tunnel: [w251] -> w27
    tunnel: [w250] -> w26
    tunnel: w5 -> [w246]
    tunnel: [w246] -> w4
    tunnel: w33 -> [w273]
    tunnel: w32 -> [w272]
    tunnel: w31 -> [w267]
    tunnel: w30 -> [w271]
    tunnel: w29 -> [w266]
    tunnel: w28 -> [w270]
    tunnel: w27 -> [w269]
    tunnel: w26 -> [w268]
    tunnel: [w273] -> w25
    tunnel: [w272] -> w24
    tunnel: [w267] -> w23
    tunnel: [w271] -> w22
    tunnel: [w265] -> w21
    tunnel: [w270] -> w20
    tunnel: [w269] -> w19
    tunnel: [w268] -> w18
    tunnel: w4 -> [w264]
    tunnel: [w264] -> w3
    tunnel: w25 -> [w291]
    tunnel: w24 -> [w290]
    tunnel: w23 -> [w285]
    tunnel: w22 -> [w284]
    tunnel: w21 -> [w289]
    tunnel: w20 -> [w288]
    tunnel: w19 -> [w287]
    tunnel: w18 -> [w286]
    tunnel: [w291] -> w17
    tunnel: [w290] -> w16
    tunnel: [w285] -> w15
    tunnel: [w283] -> w14
    tunnel: [w289] -> w13
    tunnel: [w288] -> w12
    tunnel: [w287] -> w11
    tunnel: [w286] -> w10
    tunnel: w3 -> [w282]
    tunnel: [w282] -> w2
    tunnel: w17 -> [_]
    tunnel: w16 -> [_]
    tunnel: w15 -> [_]
    tunnel: w14 -> [w302]
    tunnel: w13 -> [w303]
    tunnel: w12 -> [w304]
    tunnel: w11 -> [w305]
    tunnel: w10 -> [w306]
    tunnel: w2 -> [w301]
    tunnel: [w300] -> w1
    tunnel: w1 -> [w307]
    frame #0 {
      # "Controles."
    }
    frame #1 {
      # "\"Descomprimir\" datos."
      n2 = Unbundle By Name(w80) -> ("Recetas Allen Bradley"=w87:T2, "Recetas Schneider"=w86:T3, "Recetas Delta"=w85:T4, "Recetas ABB"=w84:T5, "Recetas LS Electric"=w83:T6)
    }
    frame #2 {
      # "Buscar índice en arreglo según fabricante."
      n3 = case shown="0, Default" w96 {
        tunnel: w95 -> [w99 _ _ _ _]
        tunnel: w90 -> [w98 w107 w115 w123 w131]
        tunnel: w94 -> [_ w105 _ _ _]
        tunnel: w93 -> [_ _ w113 _ _]
        tunnel: w92 -> [_ _ _ w121 _]
        tunnel: w91 -> [_ _ _ _ w129]
        tunnel: [w97 w106 w114 w122 w130] -> w89
        frame 0, Default {
          # "Allen Bradley."
          n4 = for {
            tunnel: w99 -> [w104] mode=indexing
            tunnel: w98 -> [w102]
            tunnel: [w101] -> w97
            tunnel: [w100] -> _
            i -> [w101]
            stop <- w100 stop-if-true
            # "Buscar en arreglo."
            n5 = Unbundle By Name(w104) -> ("Índice"=w103:u32)
            n6 = Equal?(x=w103, y=w102) -> (x = y?=w100:bool)
          }
        }
        frame 1 {
          # "Schneider."
          n7 = for {
            tunnel: w105 -> [w112] mode=indexing
            tunnel: w107 -> [w110]
            tunnel: [w109] -> w106
            tunnel: [w108] -> _
            i -> [w109]
            stop <- w108 stop-if-true
            # "Buscar en arreglo."
            n8 = Unbundle By Name(w112) -> ("Índice"=w111:u32)
            n9 = Equal?(x=w111, y=w110) -> (x = y?=w108:bool)
          }
        }
        frame 2 {
          # "Delta."
          n10 = for {
            tunnel: w113 -> [w120] mode=indexing
            tunnel: w115 -> [w118]
            tunnel: [w117] -> w114
            tunnel: [w116] -> _
            i -> [w117]
            stop <- w116 stop-if-true
            # "Buscar en arreglo."
            n11 = Unbundle By Name(w120) -> ("Índice"=w119:u32)
            n12 = Equal?(x=w119, y=w118) -> (x = y?=w116:bool)
          }
        }
        frame 3 {
          # "ABB."
          n13 = for {
            tunnel: w121 -> [w128] mode=indexing
            tunnel: w123 -> [w126]
            tunnel: [w125] -> w122
            tunnel: [w124] -> _
            i -> [w125]
            stop <- w124 stop-if-true
            # "Buscar en arreglo."
            n14 = Unbundle By Name(w128) -> ("Índice"=w127:u32)
            n15 = Equal?(x=w127, y=w126) -> (x = y?=w124:bool)
          }
        }
        frame 4 {
          # "LS Electric."
          n16 = for {
            tunnel: w129 -> [w136] mode=indexing
            tunnel: w131 -> [w134]
            tunnel: [w133] -> w130
            tunnel: [w132] -> _
            i -> [w133]
            stop <- w132 stop-if-true
            # "Buscar en arreglo."
            n17 = Unbundle By Name(w136) -> ("Índice"=w135:u32)
            n18 = Equal?(x=w135, y=w134) -> (x = y?=w132:bool)
          }
        }
      }
    }
    frame #3 {
      # "Eliminar posición de arreglo."
      n19 = case shown="0, Default" w154 {
        selector: w154 -> [w161 w174 w185 w196 w207]
        tunnel: w153 -> [w165 w169 w181 w193 w206]
        tunnel: w151 -> [w156 w168 w180 w192 w205]
        tunnel: w149 -> [w157 w170 w179 w191 w204]
        tunnel: w147 -> [w158 w171 w182 w190 w203]
        tunnel: w145 -> [w159 w172 w183 w194 w202]
        tunnel: [w163 w169 w181 w193 w206] -> w152
        tunnel: [w156 w167 w180 w192 w205] -> w150
        tunnel: [w157 w170 w178 w191 w204] -> w148
        tunnel: [w158 w171 w182 w189 w203] -> w146
        tunnel: [w159 w172 w183 w194 w201] -> w144
        tunnel: w141 -> [w162 w175 w186 w197 w208]
        tunnel: [w162 w175 w186 w197 w208] -> w143
        tunnel: [w161 w174 w185 w196 w207] -> w142
        tunnel: [w160 w173 w184 w195 w200] -> w140
        tunnel: w139 -> [w160 w173 w184 w195 w200]
        tunnel: w138 -> [w155 w166 w177 w188 w199]
        tunnel: [w155 w166 w177 w188 w199] -> w137
        frame 0, Default {
          # "Allen Bradley."
          n20 = Delete From Array(array=w165, length=1, index=w160) -> (array with subset deleted=w163:T2)  [unwired: 1 out]
        }
        frame 1 {
          # "Schneider."
          n21 = Delete From Array(array=w168, length=1, index=w173) -> (array with subset deleted=w167:T3)  [unwired: 1 out]
        }
        frame 2 {
          # "Delta."
          n22 = Delete From Array(array=w179, length=1, index=w184) -> (array with subset deleted=w178:T4)  [unwired: 1 out]
        }
        frame 3 {
          # "ABB."
          n23 = Delete From Array(array=w190, length=1, index=w195) -> (array with subset deleted=w189:T5)  [unwired: 1 out]
        }
        frame 4 {
          # "LS Electric."
          n24 = Delete From Array(array=w202, length=1, index=w200) -> (array with subset deleted=w201:T6)  [unwired: 1 out]
        }
      }
    }
    frame #4 {
      # "Modificar recetas de variadores Allen Bradley."
      n25 = for {
        tunnel: w213 -> [w224]
        tunnel: w212 -> [w227] mode=indexing
        tunnel: w212 -> [w226] mode=indexing
        tunnel: [w225] -> w211 mode=indexing
        # "Modificar índices en arreglo."
        n26 = Unbundle By Name(w227) -> ("Índice"=w222:u32)
        n27 = Greater?(x=w222, y=w224) -> (0:w223:bool)
        n28 = Decrement(x=w222) -> (x-1=w220:u32)
        n29 = Select(t=w220, s=w223, f=w222) -> (s? t:f=w221:u32)
        n30 = Bundle By Name(cluster=w226, "Índice"=w221) -> (w225:T7)
      }
    }
    frame #5 {
      # "Modificar recetas de variadores Schneider.."
      n31 = for {
        tunnel: w231 -> [w242]
        tunnel: w230 -> [w245] mode=indexing
        tunnel: w230 -> [w244] mode=indexing
        tunnel: [w243] -> w229 mode=indexing
        # "Modificar índices en arreglo."
        n32 = Unbundle By Name(w245) -> ("Índice"=w240:u32)
        n33 = Greater?(x=w240, y=w242) -> (0:w241:bool)
        n34 = Decrement(x=w240) -> (x-1=w238:u32)
        n35 = Select(t=w238, s=w241, f=w240) -> (s? t:f=w239:u32)
        n36 = Bundle By Name(cluster=w244, "Índice"=w239) -> (w243:T8)
      }
    }
    frame #6 {
      # "Modificar recetas de variadores Delta."
      n37 = for {
        tunnel: w249 -> [w260]
        tunnel: w248 -> [w263] mode=indexing
        tunnel: w248 -> [w262] mode=indexing
        tunnel: [w261] -> w247 mode=indexing
        # "Modificar índices en arreglo."
        n38 = Unbundle By Name(w263) -> ("Índice"=w258:u32)
        n39 = Greater?(x=w258, y=w260) -> (0:w259:bool)
        n40 = Decrement(x=w258) -> (x-1=w256:u32)
        n41 = Select(t=w256, s=w259, f=w258) -> (s? t:f=w257:u32)
        n42 = Bundle By Name(cluster=w262, "Índice"=w257) -> (w261:T9)
      }
    }
    frame #7 {
      # "Modificar recetas de variadores ABB."
      n43 = for {
        tunnel: w267 -> [w278]
        tunnel: w266 -> [w281] mode=indexing
        tunnel: w266 -> [w280] mode=indexing
        tunnel: [w279] -> w265 mode=indexing
        # "Modificar índices en arreglo."
        n44 = Unbundle By Name(w281) -> ("Índice"=w276:u32)
        n45 = Greater?(x=w276, y=w278) -> (0:w277:bool)
        n46 = Decrement(x=w276) -> (x-1=w274:u32)
        n47 = Select(t=w274, s=w277, f=w276) -> (s? t:f=w275:u32)
        n48 = Bundle By Name(cluster=w280, "Índice"=w275) -> (w279:T10)
      }
    }
    frame #8 {
      # "Modificar recetas de variadores LS Electric."
      n49 = for {
        tunnel: w285 -> [w296]
        tunnel: w284 -> [w299] mode=indexing
        tunnel: w284 -> [w298] mode=indexing
        tunnel: [w297] -> w283 mode=indexing
        # "Modificar índices en arreglo."
        n50 = Unbundle By Name(w299) -> ("Índice"=w294:u32)
        n51 = Greater?(x=w294, y=w296) -> (0:w295:bool)
        n52 = Decrement(x=w294) -> (x-1=w292:u32)
        n53 = Select(t=w292, s=w295, f=w294) -> (s? t:f=w293:u32)
        n54 = Bundle By Name(cluster=w298, "Índice"=w293) -> (w297:T11)
      }
    }
    frame #9 {
      # "\"Descomprimir\" datos."
      n55 = Bundle By Name(cluster=w301, "Recetas Allen Bradley"=w306, "Recetas Schneider"=w305, "Recetas Delta"=w304, "Recetas ABB"=w303, "Recetas LS Electric"=w302) -> (w300:T1)
    }
    frame #10 {
      # "Indicadores."
      "Recetas Out" <- w307
    }
  }
